vi "Mutate.VeriStandStepsProjectXML.vi"(8 "error in (no error)":errorcluster, 11 "Version Build Info":T1={"VeriStand Version"="2013 SP1", "TestStand Version"="2013", "New VS Assembly Version"="2013.0.0.0", "New TS Assembly Version"="5.1.0.226", "VeriStand Steps Version String"="14.0.5.0", "Project Paths"={"MiscHelperVIs Project Path"="", "RTSequenceVIs Project Path"="", "Set Channels Project Path"="", "TS VS Logger Project Path"="", "VeriStand.exe Install Path"="", "NI_VeristandTypes.ini File Path"="", "Workspace Path"="", "VeristandSteps.csproj File Path"="", "Silent Veristand Project Path"=""}, "New TS Interop Assembly Version"="1.2.3.4", "New TS Utility Assembly Version"="5.6.7.8", "New VS Assembly Version (GAC)"="4.0.2016.0.9.9", "dotNET .config File Paths"={"MiscHelperVIs Project .config File Path"=path "C:/Users/Public/Documents/Git-Source/VeriStand-Custom-Steps-For-TestStand/Source/LabVIEW Code/Misc/MiscHelperVIs.lvproj.config", "RT Sequence VIs Project .config File Path"=path "C:/Users/Public/Documents/Git-Source/VeriStand-Custom-Steps-For-TestStand/Source/LabVIEW Code/RT Sequence/RTSequenceVIs.lvproj.config", "Set Channels Project .config File Path"=path "C:/Users/Public/Documents/Git-Source/VeriStand-Custom-Steps-For-TestStand/Source/LabVIEW Code/Set Channels/Set Channels.lvproj.config", "TS VS Logger Project .config File Path"=path "C:/Users/Public/Documents/Git-Source/VeriStand-Custom-Steps-For-TestStand/Source/LabVIEW Code/TS VS Logger/TS VS Logger.lvproj.config", "Silent Veristand Project .config File Path"=path "C:/Users/Public/Documents/Git-Source/VeriStand-Custom-Steps-For-TestStand/Source/LabVIEW Code/VeriStand Silent Start/SilentVS.lvproj.config"}}) -> (0 "error out":errorcluster, 3 "Version Build Info":T1={"VeriStand Version"="2013 SP1", "TestStand Version"="2013", "New VS Assembly Version"="2013.0.0.0", "New TS Assembly Version"="5.1.0.226", "VeriStand Steps Version String"="14.0.5.0", "Project Paths"={"MiscHelperVIs Project Path"="", "RTSequenceVIs Project Path"="", "Set Channels Project Path"="", "TS VS Logger Project Path"="", "VeriStand.exe Install Path"="", "NI_VeristandTypes.ini File Path"="", "Workspace Path"="", "VeristandSteps.csproj File Path"="", "Silent Veristand Project Path"=""}, "New TS Interop Assembly Version"="1.2.3.4", "New TS Utility Assembly Version"="5.6.7.8", "New VS Assembly Version (GAC)"="4.0.2016.0.9.9", "dotNET .config File Paths"={"MiscHelperVIs Project .config File Path"=path "C:/Users/Public/Documents/Git-Source/VeriStand-Custom-Steps-For-TestStand/Source/LabVIEW Code/Misc/MiscHelperVIs.lvproj.config", "RT Sequence VIs Project .config File Path"=path "C:/Users/Public/Documents/Git-Source/VeriStand-Custom-Steps-For-TestStand/Source/LabVIEW Code/RT Sequence/RTSequenceVIs.lvproj.config", "Set Channels Project .config File Path"=path "C:/Users/Public/Documents/Git-Source/VeriStand-Custom-Steps-For-TestStand/Source/LabVIEW Code/Set Channels/Set Channels.lvproj.config", "TS VS Logger Project .config File Path"=path "C:/Users/Public/Documents/Git-Source/VeriStand-Custom-Steps-For-TestStand/Source/LabVIEW Code/TS VS Logger/TS VS Logger.lvproj.config", "Silent Veristand Project .config File Path"=path "C:/Users/Public/Documents/Git-Source/VeriStand-Custom-Steps-For-TestStand/Source/LabVIEW Code/VeriStand Silent Start/SilentVS.lvproj.config"}})   [LabVIEW 2014, in "VeriStand Steps Version Mutation.lvlib"]
uses:
  VeriStand Steps Version Mutation.lvlib
  Types/Version Build Information.ctl
  Types/Project Paths Cluster.ctl
  Types/dotNET Config File Paths Cluster.ctl
  <vilib>/xml/Load XML File.vi
  <vilib>/xml/Close Reference(Node).vi
  <vilib>/xml/Close Reference(NNMap).vi
  <vilib>/ni/Simple XML/_polymorphics/Create Tag - Child with Text.vi
  <vilib>/xml/NI_XML.lvlib
  <resource>/objmgr/DOMUserDefRef.rc
  <vilib>/ni/Simple XML/Simple XML.lvlib
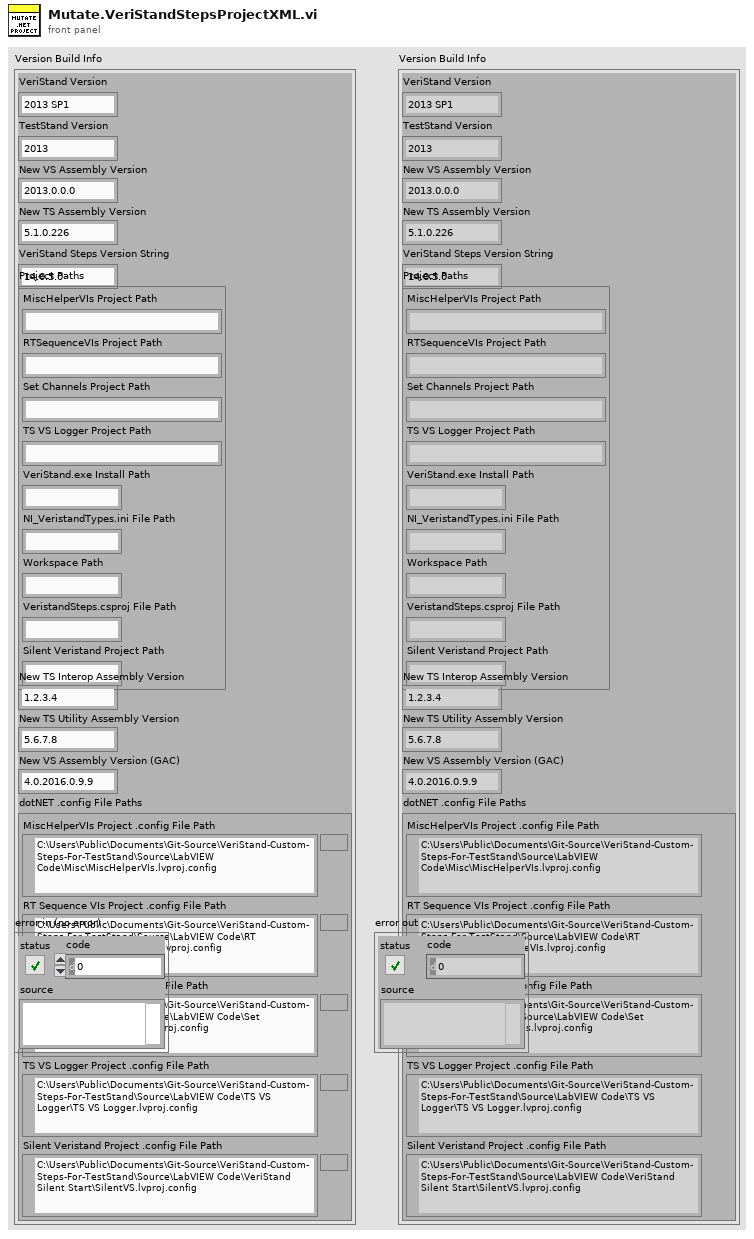
[diagram p1: front panel]
types:
  T1 = typedef "VeriStand Steps Version Mutation.lvlib/Version Build Information.ctl" = cluster{"VeriStand Version":string, "TestStand Version":string, "New VS Assembly Version":string, "New TS Assembly Version":string, "VeriStand Steps Version String":string, "Project Paths":T2, "New TS Interop Assembly Version":string, "New TS Utility Assembly Version":string, "New VS Assembly Version (GAC)":string, "dotNET .config File Paths":T3}
  T2 = typedef "VeriStand Steps Version Mutation.lvlib/Project Paths Cluster.ctl" = cluster{"MiscHelperVIs Project Path":string, "RTSequenceVIs Project Path":string, "Set Channels Project Path":string, "TS VS Logger Project Path":string, "VeriStand.exe Install Path":string, "NI_VeristandTypes.ini File Path":string, "Workspace Path":string, "VeristandSteps.csproj File Path":string, "Silent Veristand Project Path":string}
  T3 = typedef "VeriStand Steps Version Mutation.lvlib/dotNET Config File Paths Cluster.ctl" = cluster{"MiscHelperVIs Project .config File Path":path, "RT Sequence VIs Project .config File Path":path, "Set Channels Project .config File Path":path, "TS VS Logger Project .config File Path":path, "Silent Veristand Project .config File Path":path}
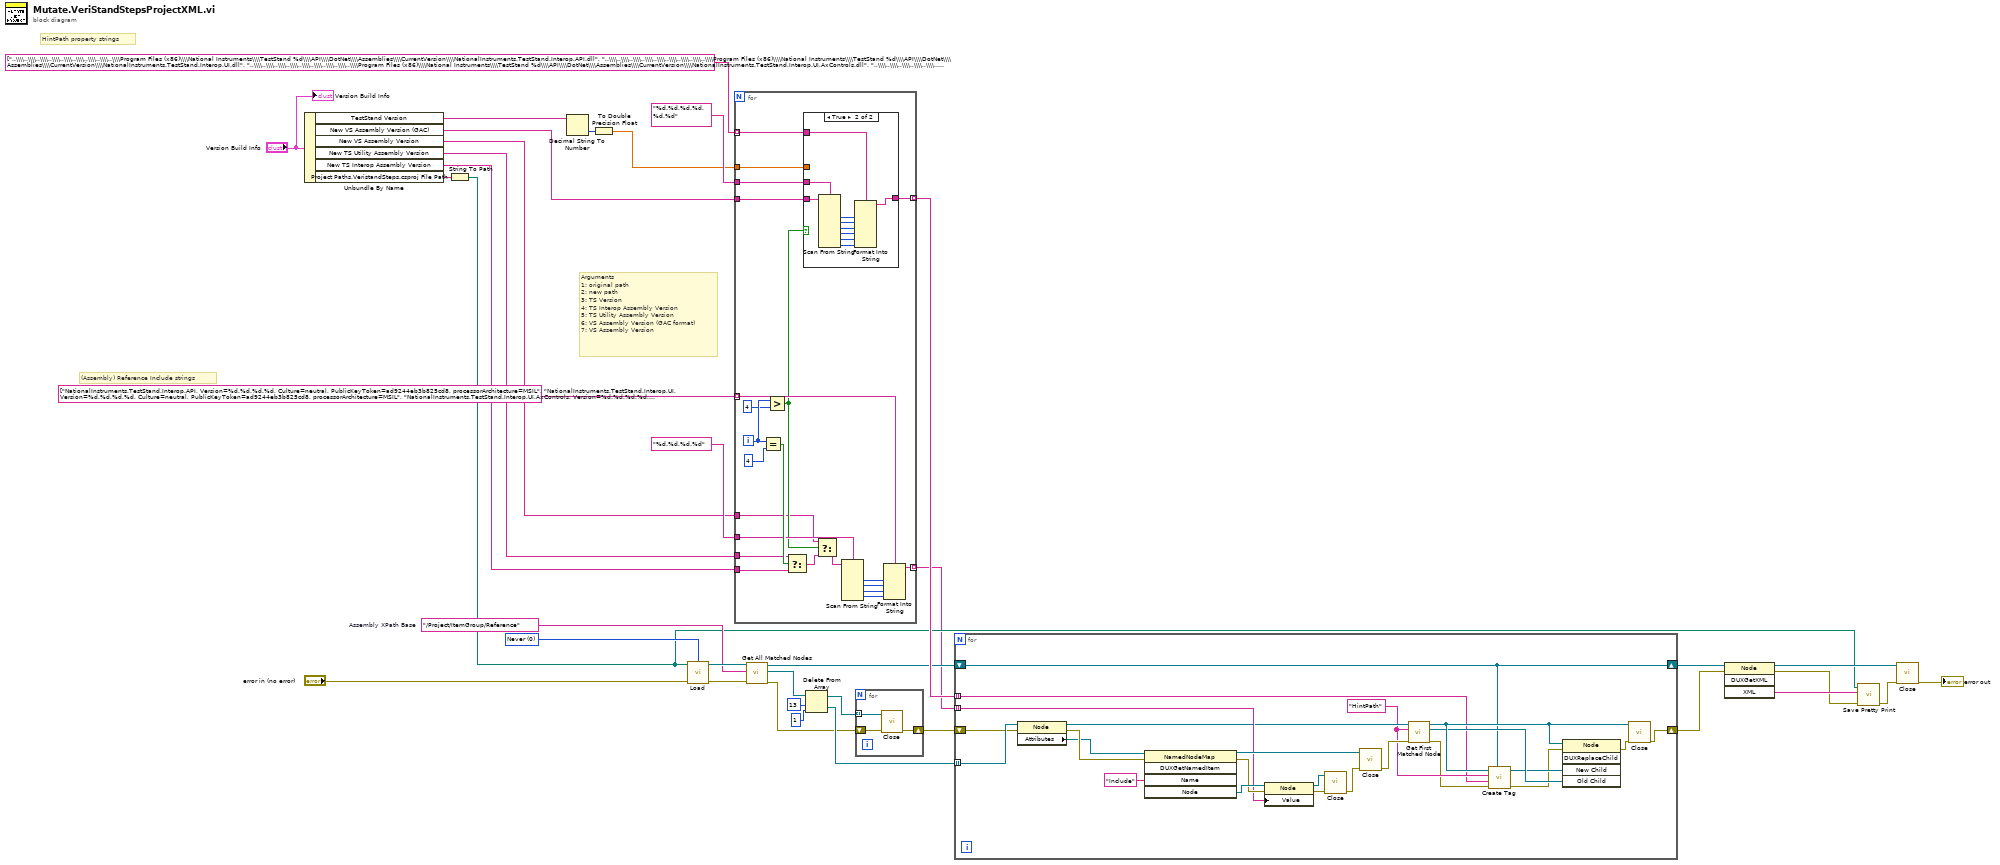
[diagram p0: block diagram]
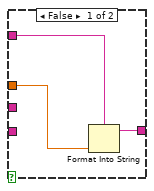
[diagram p2: hidden frame]
diagram:
  w33 = "/Project/ItemGroup/Reference"  # Assembly XPath Base
  w36 = 0 items=["Never", "Always", "Auto"] ("validate on load (Auto)")
  # "Arguments\n1: original path\n2: new path\n3: TS Version\n4: TS Interop Assembly Version\n5: TS Utility Assembly Version\n6: VS Assembly Version (GAC format)\n7: VS Assembly Version"
  # "(Assembly) Reference Include strings"
  # "HintPath property strings"
  n1 = Unbundle By Name("Version Build Info") -> ("TestStand Version"=w13:string, "New VS Assembly Version (GAC)"=w10:string, "New VS Assembly Version"=w9:string, "New TS Utility Assembly Version"=w8:string, "New TS Interop Assembly Version"=w7:string, "Project Paths.VeristandSteps.csproj File Path"=w6:string)
  n2 = String To Path(string=w6) -> (path=w5:path)
  n3 = Decimal String To Number(string=w13) -> (number=w12:i32)  [unwired: 2 in, 1 out]
  n4 = To Double Precision Float(number=w12) -> (double precision float=w11:dbl)
  n5 = call-poly <vilib>:"Load.vi"("path to XML document"=w5, "validate on load (Auto)"=w36, "error in (no error)"="error in (no error)") -> ("DOM document out"=w34:refnum<k20>, "error out"=w35:errorcluster)  [unwired: 10 in, 1 out]
  n6 = for {
    tunnel: w8 -> [w56]
    tunnel: w7 -> [w57]
    tunnel: "%d.%d.%d.%d" ("format string") -> [w55]
    tunnel: string[] ["NationalInstruments.TestStand.Interop.API, Version=%d.%d.%d.%d, Culture=neutral, PublicKeyToken=ad9244eb3b825cd8, processorArchitecture=MSIL", "NationalInstruments.TestStand.Interop.UI, Version=%d.%d.%d.%d, Culture=neutral, PublicKeyToken=ad9244eb3b825cd8, processorArchitecture=MSIL", "NationalInstruments.TestStand.Interop.UI.AxControls, Version=%d.%d.%d.%d, Culture=neutral, PublicKeyToken=ad9244eb3b825cd8, processorArchitecture=MSIL", "NationalInstruments.TestStand.Interop.UI.Support, Version=%d.%d.%d.%d, Culture=neutral, PublicKeyToken=ad9244eb3b825cd8, processorArchitecture=MSIL", "NationalInstruments.TestStand.Interop.Utility, Version=%d.%d.%d.%d, Culture=neutral, processorArchitecture=x86", "NationalInstruments.VeriStand, Version=%d.%d.%d.%d, Culture=neutral, PublicKeyToken=a6d690c380daa308, processorArchitecture=MSIL", "NationalInstruments.VeriStand.ClientAPI, Version=%d.%d.%d.%d, Culture=neutral, PublicKeyToken=a6d690c380daa308, processorArchitecture=MSIL", "NationalInstruments.VeriStand.DataTypes, Version=%d.%d.%d.%d, Culture=neutral, PublicKeyToken=a6d690c380daa308, processorArchitecture=MSIL", "NationalInstruments.VeriStand.RealTimeSequenceDefinitionApi, Version=%d.%d.%d.%d, Culture=neutral, PublicKeyToken=a6d690c380daa308, processorArchitecture=MSIL", "NationalInstruments.VeriStand.SystemDefinitionAPI, Version=%d.%d.%d.%d, Culture=neutral, PublicKeyToken=a6d690c380daa308, processorArchitecture=MSIL", "NationalInstruments.VeriStand.SystemStorage, Version=%d.%d.%d.%d, Culture=neutral, PublicKeyToken=a6d690c380daa308, processorArchitecture=MSIL", "NationalInstruments.VeriStand.SystemStorageUI, Version=%d.%d.%d.%d, Culture=neutral, PublicKeyToken=a6d690c380daa308, processorArchitecture=MSIL", "NationalInstruments.VeriStand.WorkspaceMacro, Version=%d.%d.%d.%d, Culture=neutral, PublicKeyToken=a6d690c380daa308, processorArchitecture=MSIL"] -> [w54] mode=indexing
    tunnel: [w49] -> w1 mode=indexing
    tunnel: string[] ["..\\\\..\\\\..\\\\..\\\\..\\\\..\\\\..\\\\..\\\\..\\\\Program Files (x86)\\\\National Instruments\\\\TestStand %d\\\\API\\\\DotNet\\\\Assemblies\\\\CurrentVersion\\\\NationalInstruments.TestStand.Interop.API.dll", "..\\\\..\\\\..\\\\..\\\\..\\\\..\\\\..\\\\..\\\\..\\\\Program Files (x86)\\\\National Instruments\\\\TestStand %d\\\\API\\\\DotNet\\\\Assemblies\\\\CurrentVersion\\\\NationalInstruments.TestStand.Interop.UI.dll", "..\\\\..\\\\..\\\\..\\\\..\\\\..\\\\..\\\\..\\\\..\\\\Program Files (x86)\\\\National Instruments\\\\TestStand %d\\\\API\\\\DotNet\\\\Assemblies\\\\CurrentVersion\\\\NationalInstruments.TestStand.Interop.UI.AxControls.dll", "..\\\\..\\\\..\\\\..\\\\..\\\\..\\\\..\\\\..\\\\..\\\\Program Files (x86)\\\\National Instruments\\\\TestStand %d\\\\API\\\\DotNet\\\\Assemblies\\\\CurrentVersion\\\\NationalInstruments.TestStand.Interop.UI.Support.dll", "..\\\\..\\\\..\\\\..\\\\..\\\\..\\\\..\\\\..\\\\..\\\\Program Files (x86)\\\\National Instruments\\\\TestStand %d\\\\Bin\\\\NationalInstruments.TestStand.Utility.dll", "..\\\\..\\\\..\\\\..\\\\..\\\\..\\\\..\\\\..\\\\Windows\\\\Microsoft.NET\\\\assembly\\\\GAC_MSIL\\\\NationalInstruments.VeriStand\\\\v%d.%d_%d.%d.%d.%d__a6d690c380daa308\\\\NationalInstruments.VeriStand.dll", "..\\\\..\\\\..\\\\..\\\\..\\\\..\\\\..\\\\..\\\\Windows\\\\Microsoft.NET\\\\assembly\\\\GAC_MSIL\\\\NationalInstruments.VeriStand.ClientAPI\\\\v%d.%d_%d.%d.%d.%d__a6d690c380daa308\\\\NationalInstruments.VeriStand.ClientAPI.dll", "..\\\\..\\\\..\\\\..\\\\..\\\\..\\\\..\\\\..\\\\Windows\\\\Microsoft.NET\\\\assembly\\\\GAC_MSIL\\\\NationalInstruments.VeriStand.DataTypes\\\\v%d.%d_%d.%d.%d.%d__a6d690c380daa308\\\\NationalInstruments.VeriStand.DataTypes.dll", "..\\\\..\\\\..\\\\..\\\\..\\\\..\\\\..\\\\..\\\\Windows\\\\Microsoft.NET\\\\assembly\\\\GAC_MSIL\\\\NationalInstruments.VeriStand.RealTimeSequenceDefinitionAPI\\\\v%d.%d_%d.%d.%d.%d__a6d690c380daa308\\\\NationalInstruments.VeriStand.RealTimeSequenceDefinitionAPI.dll", "..\\\\..\\\\..\\\\..\\\\..\\\\..\\\\..\\\\..\\\\Windows\\\\Microsoft.NET\\\\assembly\\\\GAC_MSIL\\\\NationalInstruments.VeriStand.SystemDefinitionAPI\\\\v%d.%d_%d.%d.%d.%d__a6d690c380daa308\\\\NationalInstruments.VeriStand.SystemDefinitionAPI.dll", "..\\\\..\\\\..\\\\..\\\\..\\\\..\\\\..\\\\..\\\\Windows\\\\Microsoft.NET\\\\assembly\\\\GAC_MSIL\\\\NationalInstruments.VeriStand.SystemStorage\\\\v%d.%d_%d.%d.%d.%d__a6d690c380daa308\\\\NationalInstruments.VeriStand.SystemStorage.dll", "..\\\\..\\\\..\\\\..\\\\..\\\\..\\\\..\\\\..\\\\Windows\\\\Microsoft.NET\\\\assembly\\\\GAC_MSIL\\\\NationalInstruments.VeriStand.SystemStorageUI\\\\v%d.%d_%d.%d.%d.%d__a6d690c380daa308\\\\NationalInstruments.VeriStand.SystemStorageUI.dll", "..\\\\..\\\\..\\\\..\\\\..\\\\..\\\\..\\\\..\\\\Windows\\\\Microsoft.NET\\\\assembly\\\\GAC_MSIL\\\\NationalInstruments.VeriStand.WorkspaceMacro\\\\v%d.%d_%d.%d.%d.%d__a6d690c380daa308\\\\NationalInstruments.VeriStand.WorkspaceMacro.dll"] -> [w48] mode=indexing
    tunnel: w11 -> [w41]
    tunnel: [w47] -> w18 mode=indexing
    tunnel: w10 -> [w43]
    tunnel: "%d.%d.%d.%d.%d.%d" ("format string") -> [w42]
    tunnel: w9 -> [w39]
    i -> [w45]
    n7 = Equal?(x=w45, y=4 ("x")) -> (x = y?=w58:bool)
    n8 = Greater?(x=w45, y=4 ("x")) -> (0:w40:bool)
    n9 = Select(t=w56, s=w58, f=w57) -> (s? t:f=w38:string)
    n10 = case shown="True" w40 {
      tunnel: w48 -> [w61 w71]
      tunnel: [w59 w70] -> w47
      tunnel: w43 -> [_ w69]
      tunnel: w42 -> [_ w68]
      tunnel: w41 -> [w60 _]
      frame False {
        n11 = Format Into String(format string=w61, w60) -> (resulting string=w59:string)  [unwired: 2 in, 1 out]
      }
      frame True {
        n12 = Scan From String(format string=w68, input string=w69) -> (output 1=w67:i32, output 2=w66:i32, output 3=w65:i32, output 4=w64:i32, output 5=w63:i32, output 6=w62:i32)  [unwired: 8 in, 3 out]
        n13 = Format Into String(format string=w71, w67, w66, w65, w64, w63, w62) -> (resulting string=w70:string)  [unwired: 2 in, 1 out]
      }
    }
    n14 = Select(t=w39, s=w40, f=w38) -> (s? t:f=w37:string)
    n15 = Scan From String(format string=w55, input string=w37) -> (output 1=w53:i32, output 2=w52:i32, output 3=w51:i32, output 4=w50:i32)  [unwired: 6 in, 3 out]
    n16 = Format Into String(format string=w54, w53, w52, w51, w50) -> (resulting string=w49:string)  [unwired: 2 in, 1 out]
  }
  n17 = call <vilib>:"Get All Matched Nodes.vi"("error in (no error)"=w35, "XPath expression"=w33, "node in"=w34) -> ("error out"=w27:errorcluster, "node result array"=w32:refnum<k20>[], "node out"=w17:refnum<k20>)  [unwired: 6 in]
  n18 = Delete From Array(array=w32, length=13, index=1 ("length")) -> (deleted portion=w29:refnum<k20>[], array with subset deleted=w28:refnum<k20>[])
  n19 = for {
    tunnel: w28 -> [w74] mode=indexing
    shift-right: [w72] -> w26
    shift-left: w27 -> [w73]
    n20 = call-poly <vilib>:"Close.vi"("error in (no error)"=w73, "node"=w74) -> ("error out"=w72:errorcluster)  [unwired: 7 in]
  }
  n21 = for {
    tunnel: w29 -> [w95] mode=indexing
    shift-right: [w89] -> w24
    shift-left: w26 -> [w94]
    tunnel: w1 -> [w88] mode=indexing
    tunnel: w18 -> [w76] mode=indexing
    shift-right: [w75] -> w16
    shift-left: w17 -> [w75]
    w83 = "HintPath" ("XPath expression")
    n22 = property class="Node"(reference=w95, error in=w94) -> (reference out=w84:refnum<k20>, error out=w98:errorcluster, "Attributes"=w96:refnum<k20>)
    n23 = invoke class="NamedNodeMap" method="DUXGetNamedItem"(reference=w96, error in=w98, "Name"="Include") -> (reference out=w90:refnum<k20>, error out=w92:errorcluster, "Node"=w93:refnum<k20>)  [unwired: 2 in, 2 out]
    n24 = property class="Node"(reference=w93, error in=w92, "Value"=w88) -> (reference out=w91:refnum<k20>, error out=w87:errorcluster)
    n25 = call-poly <vilib>:"Close.vi"("error in (no error)"=w87, "node"=w91) -> ("error out"=w86:errorcluster)  [unwired: 7 in]
    n26 = call-poly <vilib>:"Close.vi"("error in (no error)"=w86, "named node map"=w90) -> ("error out"=w85:errorcluster)  [unwired: 7 in]
    n27 = call <vilib>:"Get First Matched Node.vi"("error in (no error)"=w85, "XPath expression"=w83, "node in"=w84) -> ("error out"=w82:errorcluster, "node result"=w80:refnum<k20>, "node out"=w81:refnum<k20>)  [unwired: 6 in]
    n28 = call-poly <vilib>:"Create Tag.vi"("DOM document reference"=w75, "error in (no error)"=w82, "Text Data"=w76, "Tag Name"=w83, "Parent Element reference"=w81) -> ("error out"=w78:errorcluster, "Child Element reference"=w79:refnum<k20>)  [unwired: 5 in]
    n29 = invoke class="Node" method="DUXReplaceChild"(reference=w81, error in=w78, "New Child"=w79, "Old Child"=w80) -> (error out=w77:errorcluster)  [unwired: 1 in, 4 out]
    n30 = call-poly <vilib>:"Close.vi"("error in (no error)"=w77, "node"=w81) -> ("error out"=w89:errorcluster)  [unwired: 7 in]
  }
  n31 = invoke class="Node" method="DUXGetXML"(reference=w16, error in=w24) -> (reference out=w20:refnum<k20>, error out=w22:errorcluster, "XML"=w23:string)  [unwired: 2 in, 1 out]
  n32 = call <vilib>:"Save Pretty Print.vi"("error in (no error)"=w22, "Pretty XML String"=w23, "XML file path"=w5) -> ("error out"=w21:errorcluster)  [unwired: 7 in, 1 out]
  n33 = call-poly <vilib>:"Close.vi"("error in (no error)"=w21, "node"=w20) -> ("error out"=→"error out":errorcluster)  [unwired: 7 in]
  "Version Build Info" <- "Version Build Info"
